vi "CH1_Rx.vi"() -> ()   [LabVIEW 2018]
uses:
  Stream/Stream.lvclass
  RxTx/RxTx.lvclass
  Stream/Stream.lvclass/Stream.ctl
panel:
  in  "RxTx.lvclass":refnum<class "RxTx.lvclass">
  in  "Stream.lvclass":refnum<class "Stream.lvclass">
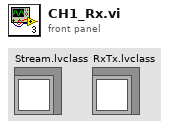
[diagram p1: front panel]
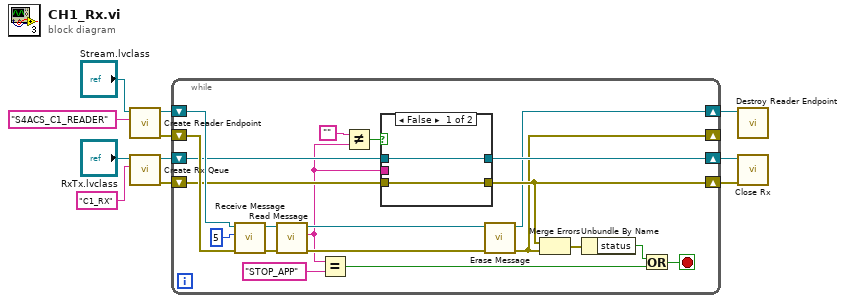
[diagram p0: block diagram]
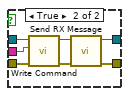
[diagram p2: hidden frame]
diagram:
  n1 = call "Create Reader Endpoint.vi"("reader name"="S4ACS_C1_READER", "Stream in"="Stream.lvclass") -> ("error out"=w8:errorcluster, "Stream out"=w9:refnum<class "Stream.lvclass">)  [unwired: 8 in]
  n2 = call "Create Rx Qeue.vi"("Reader Name"="C1_RX", "RxTx in"="RxTx.lvclass") -> ("error out"=w3:errorcluster, "RxTx out"=w4:refnum<class "RxTx.lvclass">)  [unwired: 8 in]
  n3 = while {
    shift-right: [w17] -> _
    shift-left: w8 -> [w31]
    shift-right: [w20] -> w7
    shift-left: w9 -> [w32]
    shift-right: [w24] -> w1
    shift-left: w3 -> [w28]
    shift-right: [w26] -> w2
    shift-left: w4 -> [w27]
    stop <- w14 stop-if-true
    n4 = call "Receive Message.vi"("error in (no error)"=w31, "timeout ms"=5, "Stream in"=w32) -> ("error out"=w29:errorcluster, "Stream out"=w30:refnum<class "Stream.lvclass">)  [unwired: 7 in]
    n5 = call "Read Message.vi"("error in (no error)"=w29, "Stream in"=w30) -> ("error out"=w19:errorcluster, "Message"=w16:string, "Stream out"=w18:refnum<class "Stream.lvclass">)  [unwired: 7 in]
    n6 = Equal?(x=w16, y="STOP_APP" ("reader name")) -> (x = y?=w12:bool)
    n7 = Not Equal?(x="", y=w16) -> (x != y?=w21:bool)
    n8 = case shown="False" w21 {
      tunnel: w28 -> [w33 w39]
      tunnel: w27 -> [w34 w38]
      tunnel: w16 -> [_ w37]
      tunnel: [w34 w36] -> w26
      tunnel: [w33 w35] -> w24
      frame False {
      }
      frame True {
        n9 = call "Write Command.vi"("error in (no error)"=w39, "Command"=w37, "RxTx in"=w38) -> ("error out"=w40:errorcluster, "RxTx out"=w41:refnum<class "RxTx.lvclass">)  [unwired: 7 in]
        n10 = call "Send RX Message.vi"("error in (no error)"=w40, "RxTx in"=w41) -> ("error out"=w35:errorcluster, "RxTx out"=w36:refnum<class "RxTx.lvclass">)  [unwired: 8 in]
      }
    }
    n11 = call "Erase Message.vi"("error in (no error)"=w19, "Stream in"=w18) -> ("error out"=w17:errorcluster, "Stream out"=w20:refnum<class "Stream.lvclass">)  [unwired: 8 in]
    n12 = Merge Errors(w24, w17) -> (w25:errorcluster)
    n13 = Unbundle By Name(w25) -> ("status"=w13:bool)
    n14 = Or(x=w13, y=w12) -> (x .or. y?=w14:bool)
  }
  n15 = call "Destroy Reader Endpoint.vi"("Stream in"=w7) -> ()  [unwired: 9 in, 2 out]
  n16 = call "Close Rx.vi"("error in (no error)"=w1, "RxTx in"=w2) -> ()  [unwired: 8 in, 2 out]
